vi "volumetric_scan_flexible_timing.vi"   [LabVIEW 2017]
uses:
  <vilib>/DAQmx/write.llb/DAQmx Write (Analog 2D DBL NChan NSamp).vi
  <vilib>/DAQmx/create/channels.llb/DAQmx Create Channel (AO-Voltage-Basic).vi
  <vilib>/DAQmx/configure/timing.llb/DAQmx Timing (Sample Clock).vi
  <vilib>/DAQmx/configure/trigger.llb/DAQmx Start Trigger (Digital Edge).vi
  <vilib>/DAQmx/miscellaneous.llb/DAQmx Fill In Error Info.vi
  <vilib>/DAQmx/create/channels.llb/DAQmx Create Channel (CO-Pulse Generation-Frequency).vi
  <vilib>/DAQmx/configure/timing.llb/DAQmx Timing (Implicit).vi
  <resource>/objmgr/daqmx.rc
types:
  T1 = enum32{"Invalid", "Standard", "Closed", "Hidden", "Minimized", "Maximized"}
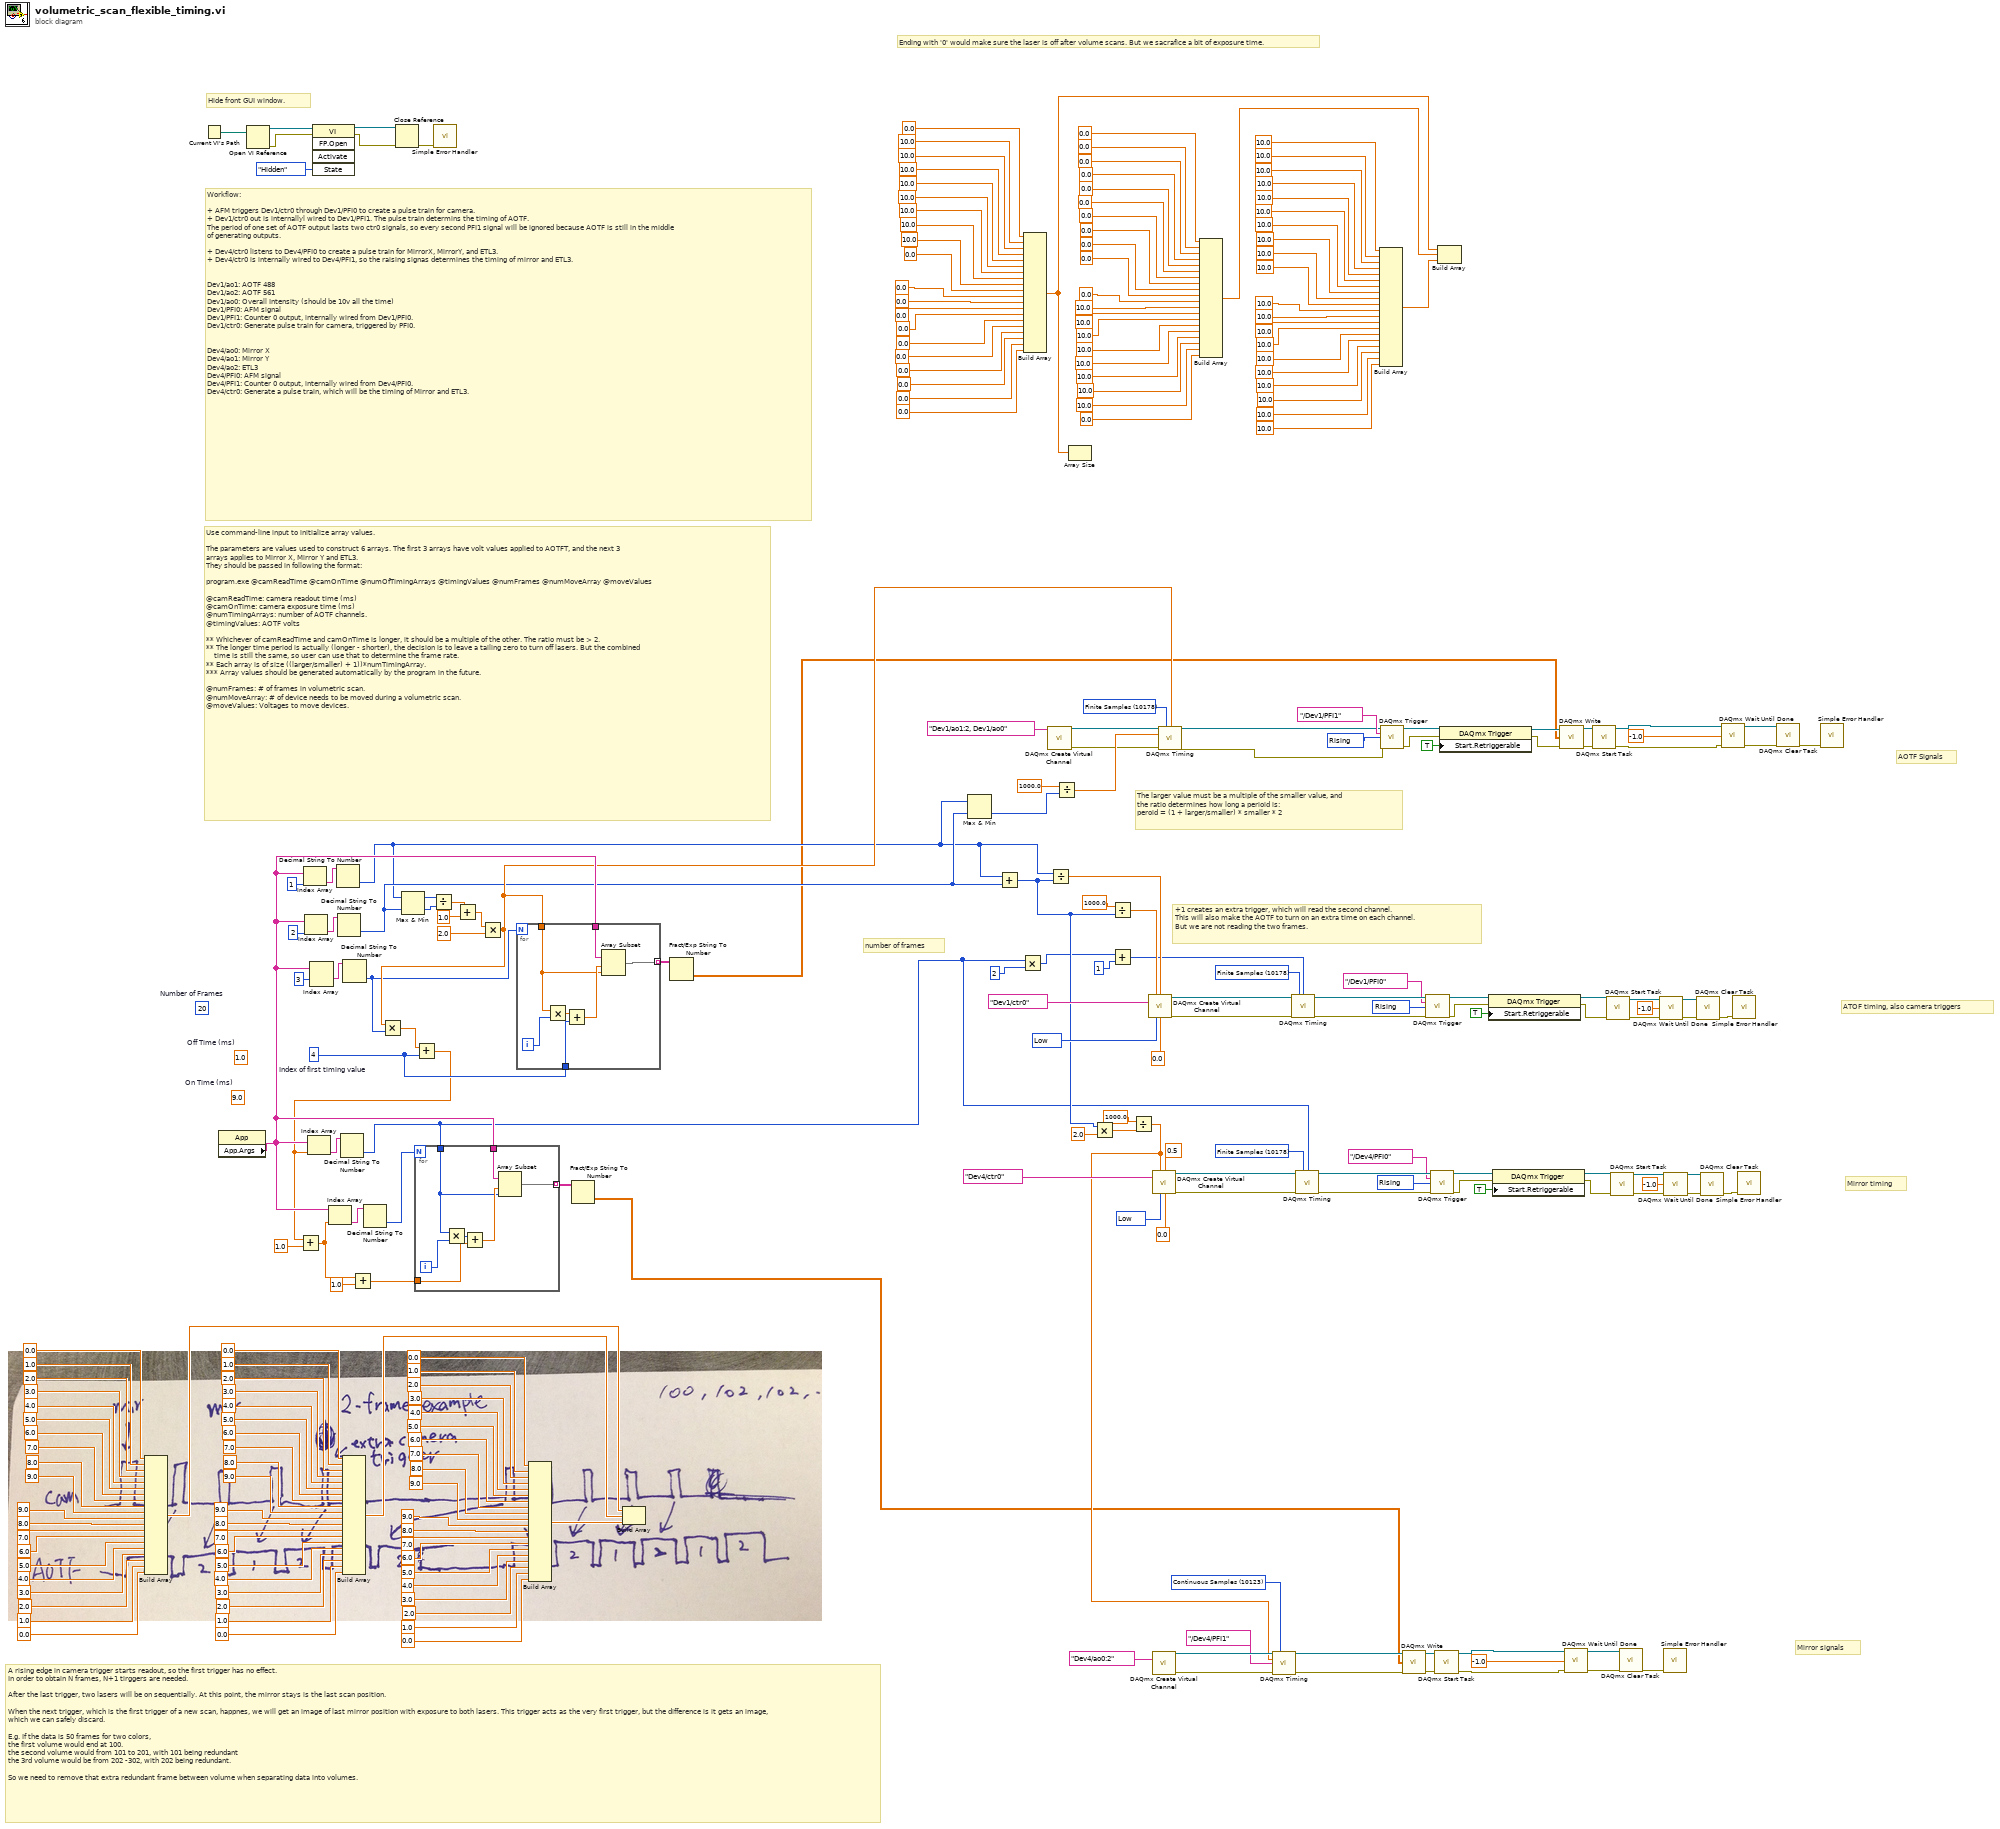
[diagram p0: block diagram]
diagram:
  w22 = 4  # Index of first timing value
  w112 = 10123 items=["Finite Samples"=10178, "Continuous Samples"=10123, "Hardware Timed Single Point"=12522] ("sample mode")
  w123 = 10178 items=["Finite Samples"=10178, "Continuous Samples"=10123, "Hardware Timed Single Point"=12522] ("sample mode")
  w124 = 10214 items=["High"=10192, "Low"=10214] ("idle state")
  w132 = 10280 items=["Rising"=10280, "Falling"=10171] ("edge")
  (unwired) 20  # Number of Frames
  w178 = 10280 items=["Rising"=10280, "Falling"=10171] ("edge")
  w190 = 10178 items=["Finite Samples"=10178, "Continuous Samples"=10123, "Hardware Timed Single Point"=12522] ("sample mode")
  (unwired) 1.0  # Off Time (ms)
  w239 = 10280 items=["Rising"=10280, "Falling"=10171] ("edge")
  w241 = 10214 items=["High"=10192, "Low"=10214] ("idle state")
  w244 = 10178 items=["Finite Samples"=10178, "Continuous Samples"=10123, "Hardware Timed Single Point"=12522] ("sample mode")
  (unwired) 9.0  # On Time (ms)
  # "Ending with '0' would make sure the laser is off after volume scans. But we sacrafice a bit of exposure time."
  # "A rising edge in camera trigger starts readout, so the first trigger has no effect.\nIn order to obtain N frames, N+1 tirggers are needed.\n\nAfter the last trigger, two lasers will be on sequentially. At this point, the mirror stays is the last scan position.\n\nWhen the next trigger, which is the first trigger of a new scan, happnes, we will get an image of last mirror position with exposure to both lasers. This trigger acts as the very first trigger, but the difference is it gets an image, \nwhich we can safely discard. \n\nE.g. If the data is 50 frames for two colors, \nthe first volume would end at 100.\nthe second volume would from 101 to 201, with 101 being redundant\nthe 3rd volume would be from 202 -302, with 202 being redundant.\n\nSo we need to remove that extra redundant frame between volume when separating data into volumes."
  # "Mirror timing"
  # "Mirror signals"
  # "ATOF timing, also camera triggers"
  # "AOTF Signals"
  # "+1 creates an extra trigger, which will read the second channel.\nThis will also make the AOTF to turn on an extra time on each channel.\nBut we are not reading the two frames."
  # "The larger value must be a multiple of the smaller value, and\nthe ratio determines how long a perioid is:\nperoid = (1 + larger/smaller) * smaller * 2"
  # "number of frames"
  # "Use command-line input to initialize array values.\n\nThe parameters are values used to construct 6 arrays. The first 3 arrays have volt values applied to AOTFT, and the next 3 \narrays applies to Mirror X, Mirror Y and ETL3.\nThey should be passed in following the format:\n\nprogram.exe @camReadTime @camOnTime @numOfTimingArrays @timingValues @numFrames @numMoveArray @moveValues\n\n@camReadTime: camera readout time (ms)\n@camOnTime: camera exposure time (ms) \n@numTimingArrays: number of AOTF channels.\n@timingValues: AOTF volts\n\n** Whichever of camReadTime and camOnTime is longer, it should be a multiple of the other. The ratio must be > 2.\n** The longer time period is actually (longer - shorter), the decision is to leave a tailing zero to turn off lasers. But the combined\n    time is still the same, so user can use that to determine the frame rate.\n** Each array is of size ((larger/smaller) + 1))*numTimingArray.\n*** Array values should be generated automatically by the program in the future.\n\n@numFrames: # of frames in volumetric scan.\n@numMoveArray: # of device needs to be moved during a volumetric scan.\n@moveValues: Voltages to move devices."
  # "Hide front GUI window."
  # "Workflow:\n\n+ AFM triggers Dev1/ctr0 through Dev1/PFI0 to create a pulse train for camera.\n+ Dev1/ctr0 out is internallyl wired to Dev1/PFI1. The pulse train determins the timing of AOTF.\nThe period of one set of AOTF output lasts two ctr0 signals, so every second PFI1 signal will be ignored because AOTF is still in the middle\nof generating outputs. \n\n+ Dev4/ctr0 listens to Dev4/PFI0 to create a pulse train for MirrorX, MirrorY, and ETL3.\n+ Dev4/ctr0 is internally wired to Dev4/PFI1, so the raising signas determines the timing of mirror and ETL3.\n\n\nDev1/ao1: AOTF 488\nDev1/ao2: AOTF 561\nDev1/ao0: Overall Intensity (should be 10v all the time)\nDev1/PFI0: AFM signal \nDev1/PFI1: Counter 0 output, internally wired from Dev1/PFI0.\nDev1/ctr0: Generate pulse train for camera, triggered by PFI0.\n\n\nDev4/ao0: Mirror X\nDev4/ao1: Mirror Y\nDev4/ao2: ETL3\nDev4/PFI0: AFM signal \nDev4/PFI1: Counter 0 output, internally wired from Dev4/PFI0.\nDev4/ctr0: Generate a pulse train, which will be the timing of Mirror and ETL3."
  n1 = Build Array(0.0 ("element"), 1.0 ("element"), 2.0 ("element"), 3.0 ("element"), 4.0 ("element"), 5.0 ("element"), 6.0 ("element"), 7.0 ("element"), 8.0 ("element"), 9.0 ("element"), 9.0 ("element"), 8.0 ("element"), 7.0 ("element"), 6.0 ("element"), 5.0 ("element"), 4.0 ("element"), 3.0 ("element"), 2.0 ("element"), 1.0 ("element"), 0.0 ("element")) -> (w59:dbl[])
  n2 = Current VI's Path() -> (path=w259:path)
  n3 = property class="App"() -> ("App.Args"=w24:string[])  [unwired: 2 in, 2 out]
  n4 = Open VI Reference(vi path=w259) -> (vi reference=w257:refnum<vi>, error out=w256:errorcluster)  [unwired: 5 in]
  n5 = Index Array(array=w24, index=1) -> (element=w33:string)
  n6 = Index Array(array=w24, index=2) -> (element=w31:string)
  n7 = Index Array(array=w24, index #1=3 ("index")) -> (element #1=w29:string)  [unwired: 1 in, 1 out]
  n8 = invoke class="VI" method="FP.Open"(reference=w257, error in=w256, "State"=T1."Hidden") -> (reference out=w255:refnum<vi>, error out=w254:errorcluster)  [unwired: 2 in, 3 out]
  n9 = Decimal String To Number(string=w33) -> (number=w8:i32)  [unwired: 2 in, 1 out]
  n10 = Decimal String To Number(string=w31) -> (number=w11:i32)  [unwired: 2 in, 1 out]
  n11 = Build Array(0.0 ("element"), 1.0 ("element"), 2.0 ("element"), 3.0 ("element"), 4.0 ("element"), 5.0 ("element"), 6.0 ("element"), 7.0 ("element"), 8.0 ("element"), 9.0 ("element"), 9.0 ("element"), 8.0 ("element"), 7.0 ("element"), 6.0 ("element"), 5.0 ("element"), 4.0 ("element"), 3.0 ("element"), 2.0 ("element"), 1.0 ("element"), 0.0 ("element")) -> (w37:dbl[])
  n12 = Decimal String To Number(string=w29) -> (number=w15:i32)  [unwired: 2 in, 1 out]
  n13 = Close Reference(reference=w255, error in (no error)=w254) -> (error out=w258:errorcluster)
  n14 = Max & Min(x=w8, y=w11) -> (max(x,y)=w10:i32, min(x,y)=w9:i32)
  n15 = Divide(x=w10, y=w9) -> (x/y=w27:dbl)
  n16 = call <vilib>:"Simple Error Handler.vi"("error in (no error)"=w258) -> ()  [unwired: 4 in, 5 out]
  n17 = Add(x=w27, y=1.0) -> (x+y=w25:dbl)
  n18 = Multiply(x=w25, y=2.0) -> (x*y=w16:dbl)
  n19 = Multiply(x=w16, y=w15) -> (x*y=w23:dbl)
  n20 = Add(x=w23, y=w22) -> (x+y=w21:dbl)
  n21 = Add(x=w21, y=1.0) -> (x+y=w19:dbl)
  n22 = Index Array(array=w24, index=w21) -> (element=w35:string)
  n23 = Index Array(array=w24, index=w19) -> (element=w36:string)
  n24 = Decimal String To Number(string=w35) -> (number=w14:i32)  [unwired: 2 in, 1 out]
  n25 = Add(x=w19, y=1.0) -> (x+y=w17:dbl)
  n26 = Decimal String To Number(string=w36) -> (number=w13:i32)  [unwired: 2 in, 1 out]
  n27 = for {
    N: w13 -> [_]
    tunnel: [w263] -> w5 mode=indexing
    tunnel: w24 -> [w262]
    tunnel: w14 -> [w261]
    tunnel: w17 -> [w260]
    i -> [w266]
    n28 = Multiply(x=w261, y=w266) -> (x*y=w265:i32)
    n29 = Add(x=w265, y=w260) -> (x+y=w264:dbl)
    n30 = Array Subset(array=w262, index=w264, length=w261) -> (w263:string[])
  }
  n31 = for {
    N: w15 -> [_]
    tunnel: [w270] -> w7 mode=indexing
    tunnel: w24 -> [w269]
    tunnel: w16 -> [w267]
    tunnel: w22 -> [w268]
    i -> [w273]
    n32 = Multiply(x=w267, y=w273) -> (x*y=w272:dbl)
    n33 = Add(x=w272, y=w268) -> (x+y=w271:dbl)
    n34 = Array Subset(array=w269, index=w271, length=w267) -> (w270:string[])
  }
  n35 = Build Array(0.0 ("element"), 1.0 ("element"), 2.0 ("element"), 3.0 ("element"), 4.0 ("element"), 5.0 ("element"), 6.0 ("element"), 7.0 ("element"), 8.0 ("element"), 9.0 ("element"), 9.0 ("element"), 8.0 ("element"), 7.0 ("element"), 6.0 ("element"), 5.0 ("element"), 4.0 ("element"), 3.0 ("element"), 2.0 ("element"), 1.0 ("element"), 0.0 ("element")) -> (w38:dbl[])
  n36 = Fract/Exp String To Number(string=w5) -> (number=w4:dbl[][])  [unwired: 3 in, 1 out]
  n37 = Build Array(w59, w37, w38) -> ()  [unwired: 1 out]
  n38 = Fract/Exp String To Number(string=w7) -> (number=w6:dbl[][])  [unwired: 3 in, 1 out]
  n39 = Max & Min(x=w8, y=w11) -> (min(x,y)=w12:i32)  [unwired: 1 out]
  n40 = Add(x=w8, y=w11) -> (x+y=w119:i32)
  n41 = Multiply(x=w14, y=2) -> (x*y=w3:i32)
  n42 = Build Array(0.0 ("element"), 10.0 ("element"), 10.0 ("element"), 10.0 ("element"), 10.0 ("element"), 10.0 ("element"), 10.0 ("element"), 10.0 ("element"), 10.0 ("element"), 0.0 ("element"), 0.0 ("element"), 0.0 ("element"), 0.0 ("element"), 0.0 ("element"), 0.0 ("element"), 0.0 ("element"), 0.0 ("element"), 0.0 ("element"), 0.0 ("element"), 0.0 ("element")) -> (w167:dbl[])
  n43 = call-poly <vilib>:"DAQmx Create Virtual Channel.vi"("physical channels"=tag "Dev1/ao1:2, Dev1/ao0") -> ("task out"=w181:refnum<k21>, "error out"=w180:errorcluster)  [unwired: 13 in]
  n44 = Divide(x=w8, y=w119) -> (x/y=w238:dbl)
  n45 = Divide(x=1000.0, y=w12) -> (x/y=w191:dbl)
  n46 = Array Size(array=w167) -> ()  [unwired: 1 out]
  n47 = Multiply(x=w119, y=2.0) -> (x*y=w118:dbl)
  n48 = Divide(x=1000.0, y=w119) -> (x/y=w193:dbl)
  n49 = Add(x=w3, y=1) -> (x+y=w1:i32)
  n50 = Divide(x=1000.0, y=w118) -> (x/y=w100:dbl)
  n51 = call-poly <vilib>:"DAQmx Create Virtual Channel.vi"("frequency"=w193, "duty cycle"=w238, "counter"=tag "Dev1/ctr0", "idle state"=w241, "initial delay"=0.0) -> ("task out"=w170:refnum<k21>, "error out"=w169:errorcluster)  [unwired: 9 in]
  n52 = call-poly <vilib>:"DAQmx Create Virtual Channel.vi"("frequency"=w100, "duty cycle"=0.5, "counter"=tag "Dev4/ctr0", "idle state"=w124, "initial delay"=0.0) -> ("task out"=w126:refnum<k21>, "error out"=w125:errorcluster)  [unwired: 9 in]
  n53 = call-poly <vilib>:"DAQmx Create Virtual Channel.vi"("physical channels"=tag "Dev4/ao0:2") -> ("task out"=w114:refnum<k21>, "error out"=w101:errorcluster)  [unwired: 13 in]
  n54 = call-poly <vilib>:"DAQmx Timing.vi"("task/channels in"=w181, "sample mode"=w190, "samples per channel"=w16, "rate"=w191, "error in"=w180) -> ("task out"=w177:refnum<k21>, "error out"=w176:errorcluster)  [unwired: 9 in]
  n55 = Build Array(0.0 ("element"), 0.0 ("element"), 0.0 ("element"), 0.0 ("element"), 0.0 ("element"), 0.0 ("element"), 0.0 ("element"), 0.0 ("element"), 0.0 ("element"), 0.0 ("element"), 0.0 ("element"), 10.0 ("element"), 10.0 ("element"), 10.0 ("element"), 10.0 ("element"), 10.0 ("element"), 10.0 ("element"), 10.0 ("element"), 10.0 ("element"), 0.0 ("element")) -> (w198:dbl[])
  n56 = call-poly <vilib>:"DAQmx Timing.vi"("task/channels in"=w114, "sample mode"=w112, "rate"=w100, "source"=tag "/Dev4/PFI1", "error in"=w101) -> ("task out"=w103:refnum<k21>, "error out"=w102:errorcluster)  [unwired: 9 in]
  n57 = call-poly <vilib>:"DAQmx Timing.vi"("task/channels in"=w170, "sample mode"=w244, "samples per channel"=w1, "error in"=w169) -> ("task out"=w250:refnum<k21>, "error out"=w251:errorcluster)  [unwired: 10 in]
  n58 = call-poly <vilib>:"DAQmx Timing.vi"("task/channels in"=w126, "sample mode"=w123, "samples per channel"=w14, "error in"=w125) -> ("task out"=w139:refnum<k21>, "error out"=w140:errorcluster)  [unwired: 10 in]
  n59 = Build Array(10.0 ("element"), 10.0 ("element"), 10.0 ("element"), 10.0 ("element"), 10.0 ("element"), 10.0 ("element"), 10.0 ("element"), 10.0 ("element"), 10.0 ("element"), 10.0 ("element"), 10.0 ("element"), 10.0 ("element"), 10.0 ("element"), 10.0 ("element"), 10.0 ("element"), 10.0 ("element"), 10.0 ("element"), 10.0 ("element"), 10.0 ("element"), 10.0 ("element")) -> (w142:dbl[])
  n60 = call-poly <vilib>:"DAQmx Trigger.vi"("task/channels in"=w177, "source"=tag "/Dev1/PFI1", "edge"=w178, "error in"=w176) -> ("task out"=w174:refnum<k21>, "error out"=w171:errorcluster)  [unwired: 10 in]
  n61 = call-poly <vilib>:"DAQmx Write.vi"("task/channels in"=w103, "data"=w4, "error in"=w102) -> ("task out"=w105:refnum<k21>, "error out"=w104:errorcluster)  [unwired: 10 in, 1 out]
  n62 = call-poly <vilib>:"DAQmx Trigger.vi"("task/channels in"=w250, "source"=tag "/Dev1/PFI0", "edge"=w239, "error in"=w251) -> ("task out"=w236:refnum<k21>, "error out"=w234:errorcluster)  [unwired: 10 in]
  n63 = call-poly <vilib>:"DAQmx Trigger.vi"("task/channels in"=w139, "source"=tag "/Dev4/PFI0", "edge"=w132, "error in"=w140) -> ("task out"=w131:refnum<k21>, "error out"=w129:errorcluster)  [unwired: 10 in]
  n64 = call <vilib>:"DAQmx Start Task.vi"("task/channels in"=w105, "error in"=w104) -> ("task out"=w107:refnum<k21>, "error out"=w108:errorcluster)  [unwired: 12 in]
  n65 = Build Array(w167, w198, w142) -> ()  [unwired: 1 out]
  n66 = property class="DAQmx Trigger"(reference=w174, error in=w171, "Start.Retriggerable"=TRUE) -> (reference out=w173:refnum<k21>, error out=w172:errorcluster)
  n67 = property class="DAQmx Trigger"(reference=w236, error in=w234, "Start.Retriggerable"=TRUE) -> (reference out=w235:refnum<k21>, error out=w233:errorcluster)
  n68 = property class="DAQmx Trigger"(reference=w131, error in=w129, "Start.Retriggerable"=TRUE) -> (reference out=w130:refnum<k21>, error out=w128:errorcluster)
  n69 = call-poly <vilib>:"DAQmx Write.vi"("task/channels in"=w173, "data"=w6, "error in"=w172) -> ("task out"=w184:refnum<k21>, "error out"=w183:errorcluster)  [unwired: 10 in, 1 out]
  n70 = call <vilib>:"DAQmx Wait Until Done.vi"("task/channels in"=w107, "timeout (sec)"=-1.0, "error in"=w108) -> ("task out"=w110:refnum<k21>, "error out"=w109:errorcluster)  [unwired: 11 in]
  n71 = call <vilib>:"DAQmx Start Task.vi"("task/channels in"=w184, "error in"=w183) -> ("task out"=w186:refnum<k21>, "error out"=w187:errorcluster)  [unwired: 12 in]
  n72 = call <vilib>:"DAQmx Start Task.vi"("task/channels in"=w235, "error in"=w233) -> ("task out"=w245:refnum<k21>, "error out"=w246:errorcluster)  [unwired: 12 in]
  n73 = call <vilib>:"DAQmx Start Task.vi"("task/channels in"=w130, "error in"=w128) -> ("task out"=w134:refnum<k21>, "error out"=w135:errorcluster)  [unwired: 12 in]
  n74 = call <vilib>:"DAQmx Clear Task.vi"("task in"=w110, "error in"=w109) -> ("error out"=w111:errorcluster)  [unwired: 13 in]
  n75 = call <vilib>:"DAQmx Wait Until Done.vi"("task/channels in"=w245, "timeout (sec)"=-1.0, "error in"=w246) -> ("task out"=w248:refnum<k21>, "error out"=w247:errorcluster)  [unwired: 11 in]
  n76 = call <vilib>:"Simple Error Handler.vi"("error in (no error)"=w111) -> ()  [unwired: 4 in, 5 out]
  n77 = call <vilib>:"DAQmx Wait Until Done.vi"("task/channels in"=w134, "timeout (sec)"=-1.0, "error in"=w135) -> ("task out"=w137:refnum<k21>, "error out"=w136:errorcluster)  [unwired: 11 in]
  n78 = call <vilib>:"DAQmx Clear Task.vi"("task in"=w248, "error in"=w247) -> ("error out"=w252:errorcluster)  [unwired: 13 in]
  n79 = call <vilib>:"DAQmx Clear Task.vi"("task in"=w137, "error in"=w136) -> ("error out"=w141:errorcluster)  [unwired: 13 in]
  n80 = call <vilib>:"DAQmx Wait Until Done.vi"("task/channels in"=w186, "timeout (sec)"=-1.0, "error in"=w187) -> ("task out"=w189:refnum<k21>, "error out"=w188:errorcluster)  [unwired: 11 in]
  n81 = call <vilib>:"Simple Error Handler.vi"("error in (no error)"=w252) -> ()  [unwired: 4 in, 5 out]
  n82 = call <vilib>:"Simple Error Handler.vi"("error in (no error)"=w141) -> ()  [unwired: 4 in, 5 out]
  n83 = call <vilib>:"DAQmx Clear Task.vi"("task in"=w189, "error in"=w188) -> ("error out"=w231:errorcluster)  [unwired: 13 in]
  n84 = call <vilib>:"Simple Error Handler.vi"("error in (no error)"=w231) -> ()  [unwired: 4 in, 5 out]
